vi "SwissSPAD Live_Get FLI Parameters for HDF5.vi"(8 "error in (no error)":errorcluster) -> (0 "error out":errorcluster, 2 "# Sets":u32, 3 "Acquisition Parameters":T1, 4 "Metadata String":string)   [LabVIEW 2021]
uses:
  Phasor/Fluorescence Lifetime Parameters v3.ctl
  SwissSPAD Live_Settings List.ctl
  SwissSPAD Live_SSx PCB Version.ctl
  SwissSPAD Live_SS2 DAQ Parameters 3.ctl
  SwissSPAD Live_SS2 Gate Definition.ctl
  SwissSPAD Live_Gate Configuration Action.ctl
  SwissSPAD Live_SS2 Gate Configuration.ctl
  SwissSPAD Live_SS3 DAQ Parameters.ctl
  SwissSPAD Live_SS3 Gate Definition.ctl
  SS3 Gate Width Definition Mode.ctl
  Phasor/Fluorescence Lifetime Parameters v2.ctl
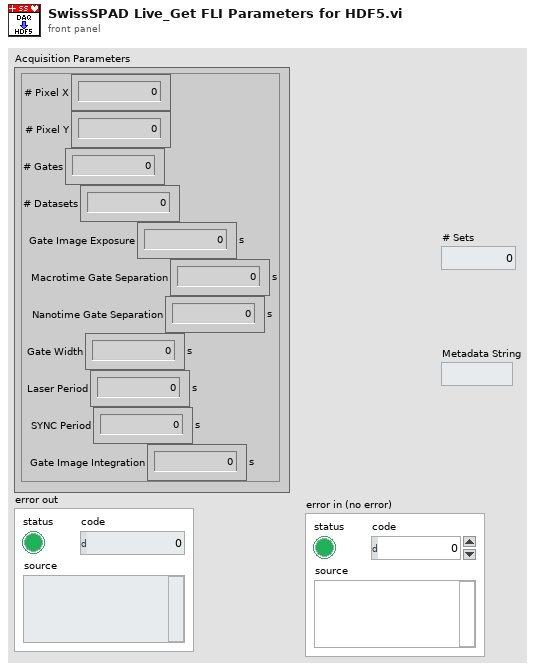
[diagram p1: front panel]
types:
  T1 = typedef "Fluorescence Lifetime Parameters v3.ctl" = cluster{"# Pixel X":i32, "# Pixel Y":i32, "# Gates":i32, "# Datasets":i32, "Gate Image Exposure":dbl[unit], "Macrotime Gate Separation":dbl[unit], "Nanotime Gate Separation":dbl[unit], "Gate Width":dbl[unit], "Laser Period":dbl[unit], "SYNC Period":dbl[unit], "Gate Image Integration":dbl[unit]}
  T2 = typedef "SwissSPAD Live_SSx PCB Version.ctl" = enum16{"unknown", "SS2 PCB1", "SS2 PCB2", "SS3 PCB1"}
  T3 = typedef "SwissSPAD Live_Settings List.ctl" = enum16{"FPGA:Bottom Half", "FPGA:Top Half", "FPGA:Bottom Bitfile Path", "FPGA:Top Bitfile Path", "FPGA:Bottom Bitstream Version", "FPGA:Top Bitstream Version", "FPGA:Auto Reset FPGA", "FPGA:Bottom FPGA Serial Number", "FPGA:Top FPGA Serial Number", "FPGA:Detector PCB Version", "Acquisition Parameters:Microlens", "Acquisition Parameters:SS2 DAQ Parameters", "Acquisition Parameters:Gate Configuration Array", "Acquisition Parameters:SS3 DAQ Parameters", "Acquisition Parameters:Buffer Size (# 8-bit Gates)", "File Information:File Information", "File Information:# Datasets in Series", "File Information:Scrambled File Flag", "File Information:SS3 Gate Slip Correction", "File Information:SS3 Hot Pixel Mismatch Detection", "File Information:Delay between Datasets", "File Information:Save Sum of All Gates Preview", "Image Parameters:Image ROI Information", "Image Parameters:Image Binning Options", "Image Parameters:SS3 Displayed Image", "Image Parameters:Image Display Options", "Image Parameters:Use Histogram Cursors", "Image Parameter:FPGA Data to Display", "UI Settings:Histogram Bins Number", "UI Settings:Use Image Display Options", "UI Settings:Verbose Settings", "UI Settings:Verbose Saving"}
  T4 = typedef "SwissSPAD Live_SS2 Gate Configuration.ctl" = cluster{"Gate Configuration":string, "Gate Offset":u32, "Gate Definition":T5}
  T5 = typedef "SwissSPAD Live_SS2 Gate Definition.ctl" = cluster{"gs_psincdec_0":u32, "gs_psincdec_1":u32, "gs_psincdec_2":u32, "gs_psincdec_3":u32, "gs_no_shift_adj_1":u32, "gs_no_shift_adj_2":u32, "gs_no_shift_adj_3":u32}
  T6 = typedef "SwissSPAD Live_Gate Configuration Action.ctl" = enum16{"Get Gate Configuration Name", "Get Configuration by Name", "Add Gate Configuration", "Delete Gate Configuration", "Rename Gate Configuration"}
  T7 = typedef "SwissSPAD Live_SS2 DAQ Parameters 3.ctl" = cluster{"10 bits":bool, "# Exposure Sequences":u32, "# 1-bit Frame per Gate":u32, "Gate Shift":u32, "# Gates per Set":u32, "# Sets":u32, "Laser Period":dbl[unit], "Sync Period":dbl[unit], "Gate Offset":u32, "Auto-adjust Gate Offset":bool, "Gate Definition":T5, "Reversed Shift":bool}
  T8 = typedef "Fluorescence Lifetime Parameters v2.ctl" = cluster{"# Pixel X":i32, "# Pixel Y":i32, "# Gates":i32, "# Datasets":i32, "Exposure/Gate":dbl[unit], "Macrotime Gate Separation":dbl[unit], "Nanotime Gate Separation":dbl[unit], "Gate Duration":dbl[unit], "Laser Period":dbl[unit], "SYNC Period":dbl[unit]}
  T9 = typedef "SwissSPAD Live_SS3 DAQ Parameters.ctl" = cluster{"10 bits":bool, "# Exposure Sequences":u32, "# 1-bit Frame per Gate":u32, "Gate Shift":u32, "# Gate Pairs per Set":u32, "# Sets":u32, "Laser Period":dbl[unit], "Sync Period":dbl[unit], "Gate Offset":u32, "Auto-adjust Gate Offset":bool, "Gate Definition":T10, "Gate Width (ns)":dbl, "Reversed Shift":bool, "Intensity Mode":bool, "Gate Definition Mode":T11}
  T10 = typedef "SwissSPAD Live_SS3 Gate Definition.ctl" = cluster{"gs_psincdec_0":u32, "gs_psincdec_1":u32, "gs_no_shift_adj_1":u32, "gate_adj_2":u32}
  T11 = typedef "SS3 Gate Width Definition Mode.ctl" = enum32{"Item 0", "Item 1"}
  T12 = typedef "SwissSPAD Live_Gate Characteristics.ctl" = cluster{"Predicted Gate Width":dbl[unit], "Gate Image Integration":dbl[unit], "Gate Image Exposure":dbl[unit], "Gate Shift":dbl[unit], "Gate Images Span":dbl[unit]}
  T13 = cluster{"Predicted Gate Width":dbl, "Gate Image Integration":dbl, "Gate Image Exposure":dbl, "Gate Shift":dbl, "Gate Images Span":dbl}
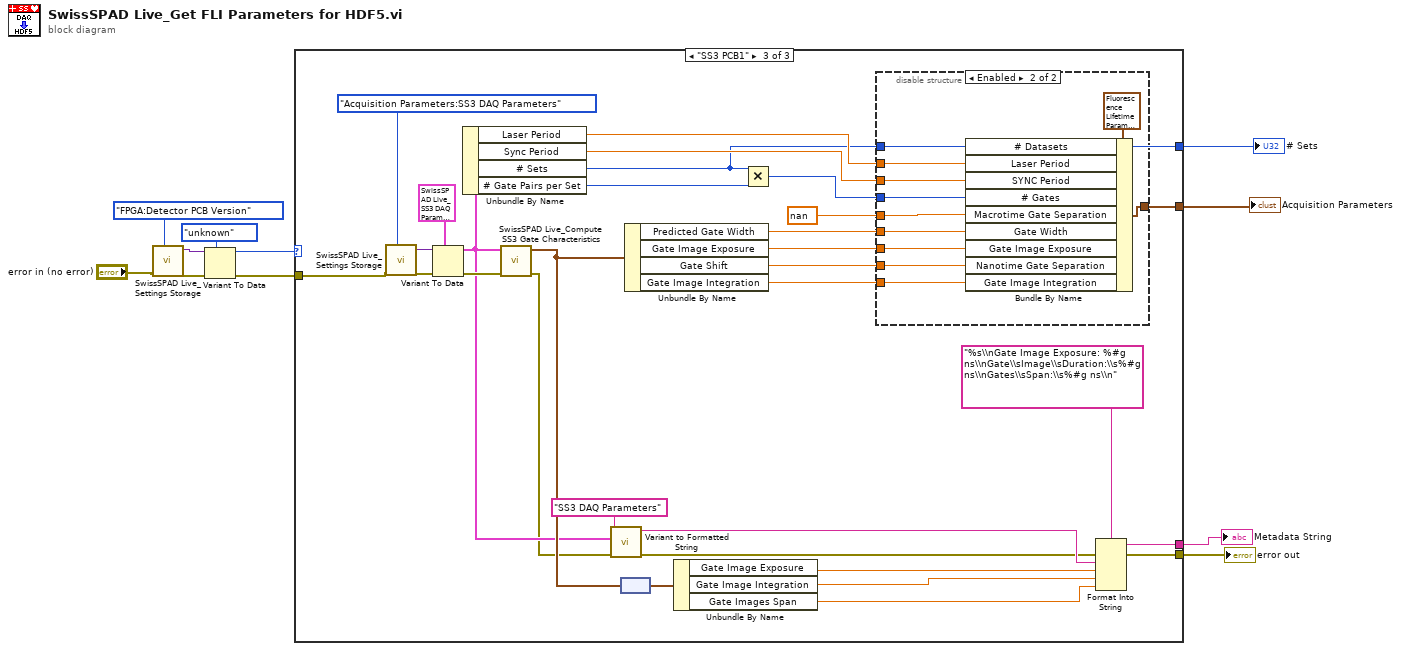
[diagram p0: block diagram]
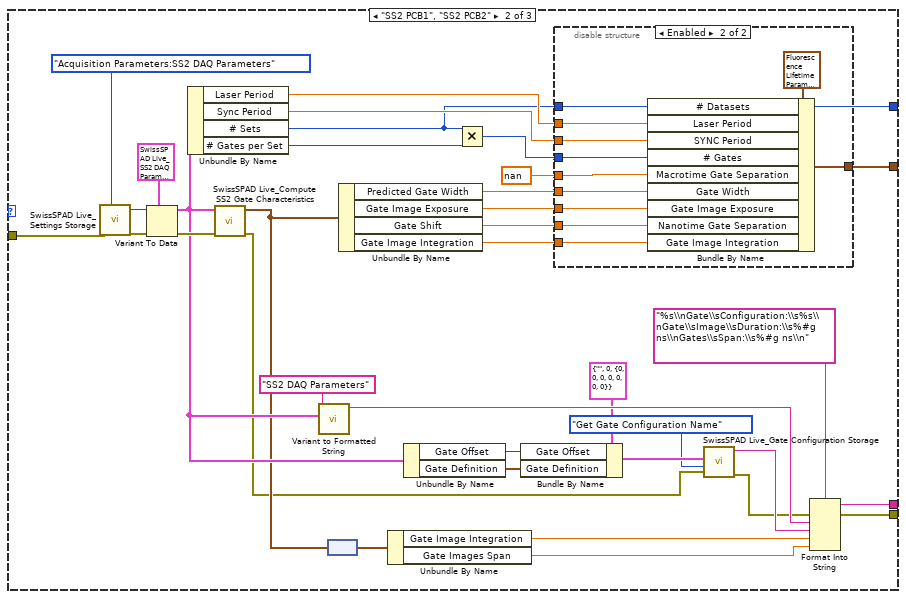
[diagram p3: hidden frame]
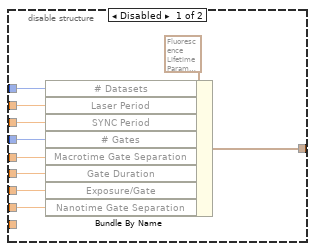
[diagram p4: hidden frame]
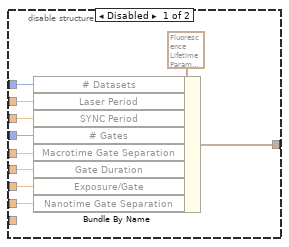
[diagram p5: hidden frame]
diagram:
  n1 = call "SwissSPAD Live_Settings Storage.vi"("Settings List"=SwissSPAD_Live_Settings_List."FPGA:Detector PCB Version", "Error In"="error in (no error)") -> ("Error Out"=w6:errorcluster, "Variant Data out"=w2:variant)  [unwired: 8 in]
  n2 = Variant To Data(error in=w6, type=SwissSPAD_Live_SSx_PCB_Version."unknown" ("Detector PCB Version"), Variant=w2) -> (data=w5:T2, error out=w4:errorcluster)
  n3 = case shown="\"SS3 PCB1\"" w5 {
    tunnel: [_ w47 w98] -> w11
    tunnel: [_ w46 w97] -> w10
    tunnel: [_ w17 w74] -> w9
    tunnel: w4 -> [w12 w19 w79]
    tunnel: [w12 w18 w75] -> w3
    frame "unknown", Default {
    }
    frame "SS2 PCB1", "SS2 PCB2" {
      n4 = call "SwissSPAD Live_Settings Storage.vi"("Settings List"=SwissSPAD_Live_Settings_List."Acquisition Parameters:SS2 DAQ Parameters", "Error In"=w19) -> ("Error Out"=w22:errorcluster, "Variant Data out"=w16:variant)  [unwired: 8 in]
      n5 = Variant To Data(error in=w22, type=T7 {"10 bits"=FALSE, "# Exposure Sequences"=0, "# 1-bit Frame per Gate"=0, "Gate Shift"=0, "# Gates per Set"=0, "# Sets"=1, "Laser Period"=0.0, "Sync Period"=0.0, "Gate Offset"=0, "Auto-adjust Gate Offset"=FALSE, "Gate Definition"={"gs_psincdec_0"=0, "gs_psincdec_1"=0, "gs_psincdec_2"=0, "gs_psincdec_3"=0, "gs_no_shift_adj_1"=0, "gs_no_shift_adj_2"=0, "gs_no_shift_adj_3"=0}, "Reversed Shift"=FALSE} ("SS2 DAQ Parameters"), Variant=w16) -> (data=w33:T7, error out=w39:errorcluster)
      n6 = Unbundle By Name(w33) -> ("Laser Period"=w29:dbl[unit], "Sync Period"=w40:dbl[unit], "# Sets"=w17:u32, "# Gates per Set"=w24:u32)
      n7 = call "SwissSPAD Live_Compute SS2 Gate Characteristics.vi"("Error In"=w39, "SS2 DAQ Parameters"=w33) -> ("Error Out"=w20:errorcluster, "Gate Characteristics"=w31:T12)  [unwired: 8 in]
      n8 = call "Variant to Formatted String.vi"("Variant"=w33, "Label"="SS2 DAQ Parameters") -> ("String"=w42:string)  [unwired: 8 in, 1 out]
      n9 = node(w31) -> (w14:T13)
      n10 = Unbundle By Name(w31) -> ("Predicted Gate Width"=w27:dbl[unit], "Gate Image Exposure"=w28:dbl[unit], "Gate Shift"=w30:dbl[unit], "Gate Image Integration"=w13:dbl[unit])
      n11 = Unbundle By Name(w14) -> ("Gate Image Integration"=w44:dbl, "Gate Images Span"=w45:dbl)
      n12 = Unbundle By Name(w33) -> ("Gate Offset"=w36:u32, "Gate Definition"=w37:T5)
      n13 = Multiply(x=w17, y=w24) -> (x*y=w25:u32)
      n14 = Bundle By Name(cluster=T4 {"Gate Configuration"="", "Gate Offset"=0, "Gate Definition"={"gs_psincdec_0"=0, "gs_psincdec_1"=0, "gs_psincdec_2"=0, "gs_psincdec_3"=0, "gs_no_shift_adj_1"=0, "gs_no_shift_adj_2"=0, "gs_no_shift_adj_3"=0}} ("Gate Configuration Definition in"), "Gate Offset"=w36, "Gate Definition"=w37) -> (w38:T4)
      n15 = disable-structure shown="Enabled" {
        disable-tunnel: [w57 w68] -> w47
        disable-tunnel: w40 -> [w56 w60]
        disable-tunnel: w30 -> [w55 w61]
        disable-tunnel: w29 -> [w54 w67]
        disable-tunnel: w28 -> [w53 w59]
        disable-tunnel: w27 -> [w52 w66]
        disable-tunnel: dbl[unit] nan ("Macrotime Gate Separation") -> [w51 w65]
        disable-tunnel: w25 -> [w50 w64]
        disable-tunnel: w17 -> [w48 w62]
        disable-tunnel: w13 -> [_ w58]
        frame Disabled {
          n16 = Bundle By Name(cluster=T8 {"# Pixel X"=0, "# Pixel Y"=0, "# Gates"=0, "# Datasets"=0, "Exposure/Gate"=0.0, "Macrotime Gate Separation"=0.0, "Nanotime Gate Separation"=0.0, "Gate Duration"=0.0, "Laser Period"=0.0, "SYNC Period"=0.0} ("FLI Parameters"), "# Datasets"=w48, "Laser Period"=w54, "SYNC Period"=w56, "# Gates"=w50, "Macrotime Gate Separation"=w51, "Gate Duration"=w52, "Exposure/Gate"=w53, "Nanotime Gate Separation"=w55) -> (w57:T8)
        }
        frame Enabled {
          n17 = Bundle By Name(cluster=T1 {"# Pixel X"=0, "# Pixel Y"=0, "# Gates"=0, "# Datasets"=0, "Gate Image Exposure"=0.0, "Macrotime Gate Separation"=0.0, "Nanotime Gate Separation"=0.0, "Gate Width"=0.0, "Laser Period"=0.0, "SYNC Period"=0.0, "Gate Image Integration"=0.0} ("FLI Parameters"), "# Datasets"=w62, "Laser Period"=w67, "SYNC Period"=w60, "# Gates"=w64, "Macrotime Gate Separation"=w65, "Gate Width"=w66, "Gate Image Exposure"=w59, "Nanotime Gate Separation"=w61, "Gate Image Integration"=w58) -> (w68:T1)
        }
      }
      n18 = call "SwissSPAD Live_Gate Configuration Storage.vi"("Error In"=w20, "Action"=SwissSPAD_Live_Gate_Configuration_Action."Get Gate Configuration Name", "Gate Configuration Definition in"=w38) -> ("Error Out"=w21:errorcluster, "Gate Configuration Name out"=w43:string)  [unwired: 3 in, 4 out]
      n19 = Format Into String(format string="%s\\nGate\\sConfiguration:\\s%s\\nGate\\sImage\\sDuration:\\s%#g ns\\nGates\\sSpan:\\s%#g ns\\n", error in=w21, w42, w43, w44, w45) -> (resulting string=w46:string, error out=w18:errorcluster)  [unwired: 1 in]
    }
    frame "SS3 PCB1" {
      n20 = call "SwissSPAD Live_Settings Storage.vi"("Settings List"=SwissSPAD_Live_Settings_List."Acquisition Parameters:SS3 DAQ Parameters", "Error In"=w79) -> ("Error Out"=w80:errorcluster, "Variant Data out"=w73:variant)  [unwired: 8 in]
      n21 = Variant To Data(error in=w80, type=T9 {"10 bits"=FALSE, "# Exposure Sequences"=0, "# 1-bit Frame per Gate"=0, "Gate Shift"=0, "# Gate Pairs per Set"=0, "# Sets"=1, "Laser Period"=0.0, "Sync Period"=0.0, "Gate Offset"=0, "Auto-adjust Gate Offset"=FALSE, "Gate Definition"={"gs_psincdec_0"=0, "gs_psincdec_1"=0, "gs_no_shift_adj_1"=0, "gate_adj_2"=0}, "Gate Width (ns)"=0.0, "Reversed Shift"=FALSE, "Intensity Mode"=FALSE, "Gate Definition Mode"=enum."Item 0"} ("SS3 DAQ Parameters"), Variant=w73) -> (data=w78:T9, error out=w91:errorcluster)
      n22 = Unbundle By Name(w78) -> ("Laser Period"=w87:dbl[unit], "Sync Period"=w92:dbl[unit], "# Sets"=w74:u32, "# Gate Pairs per Set"=w82:u32)
      n23 = call "SwissSPAD Live_Compute SS3 Gate Characteristics.vi"("Error In"=w91, "SS3 DAQ Parameters"=w78) -> ("Error Out"=w77:errorcluster, "Gate Characteristics"=w89:T12)  [unwired: 8 in]
      n24 = call "Variant to Formatted String.vi"("Error In"=w77, "Variant"=w78, "Label"="SS3 DAQ Parameters") -> ("Error Out"=w76:errorcluster, "String"=w94:string)  [unwired: 7 in]
      n25 = node(w89) -> (w69:T13)
      n26 = Unbundle By Name(w89) -> ("Predicted Gate Width"=w85:dbl[unit], "Gate Image Exposure"=w86:dbl[unit], "Gate Shift"=w88:dbl[unit], "Gate Image Integration"=w71:dbl[unit])
      n27 = Unbundle By Name(w69) -> ("Gate Image Exposure"=w70:dbl, "Gate Image Integration"=w95:dbl, "Gate Images Span"=w96:dbl)
      n28 = Multiply(x=w74, y=w82) -> (x*y=w83:u32)
      n29 = disable-structure shown="Enabled" {
        disable-tunnel: [w108 w119] -> w98
        disable-tunnel: w92 -> [w107 w118]
        disable-tunnel: w88 -> [w106 w111]
        disable-tunnel: w87 -> [w105 w112]
        disable-tunnel: w86 -> [w104 w110]
        disable-tunnel: w85 -> [w103 w117]
        disable-tunnel: dbl[unit] nan ("Macrotime Gate Separation") -> [w102 w116]
        disable-tunnel: w83 -> [w101 w115]
        disable-tunnel: w74 -> [w99 w113]
        disable-tunnel: w71 -> [_ w109]
        frame Disabled {
          n30 = Bundle By Name(cluster=T8 {"# Pixel X"=0, "# Pixel Y"=0, "# Gates"=0, "# Datasets"=0, "Exposure/Gate"=0.0, "Macrotime Gate Separation"=0.0, "Nanotime Gate Separation"=0.0, "Gate Duration"=0.0, "Laser Period"=0.0, "SYNC Period"=0.0} ("FLI Parameters"), "# Datasets"=w99, "Laser Period"=w105, "SYNC Period"=w107, "# Gates"=w101, "Macrotime Gate Separation"=w102, "Gate Duration"=w103, "Exposure/Gate"=w104, "Nanotime Gate Separation"=w106) -> (w108:T8)
        }
        frame Enabled {
          n31 = Bundle By Name(cluster=T1 {"# Pixel X"=0, "# Pixel Y"=0, "# Gates"=0, "# Datasets"=0, "Gate Image Exposure"=0.0, "Macrotime Gate Separation"=0.0, "Nanotime Gate Separation"=0.0, "Gate Width"=0.0, "Laser Period"=0.0, "SYNC Period"=0.0, "Gate Image Integration"=0.0} ("FLI Parameters"), "# Datasets"=w113, "Laser Period"=w112, "SYNC Period"=w118, "# Gates"=w115, "Macrotime Gate Separation"=w116, "Gate Width"=w117, "Gate Image Exposure"=w110, "Nanotime Gate Separation"=w111, "Gate Image Integration"=w109) -> (w119:T1)
        }
      }
      n32 = Format Into String(format string="%s\\nGate Image Exposure: %#g ns\\nGate\\sImage\\sDuration:\\s%#g ns\\nGates\\sSpan:\\s%#g ns\\n", error in=w76, w94, w70, w95, w96) -> (resulting string=w97:string, error out=w75:errorcluster)  [unwired: 1 in]
    }
  }
  "Acquisition Parameters" <- w11
  "Metadata String" <- w10
  "error out" <- w3
  "# Sets" <- w9
